vi "主程序.vi"() -> ()   [LabVIEW 2016]
panel:
  out "数值":dbl
  out "布尔":bool
  out "数字(0-1)":dbl
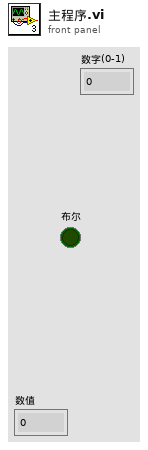
[diagram p1: front panel]
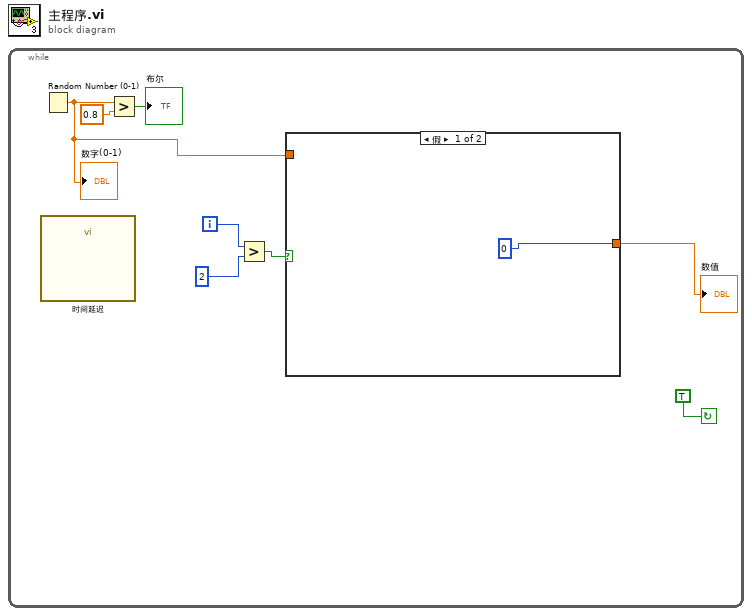
[diagram p0: block diagram]
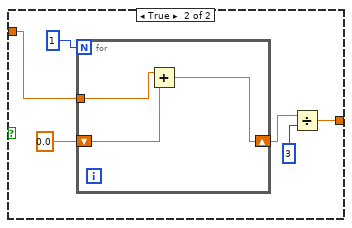
[diagram p2: hidden frame]
diagram:
  n1 = while {
    i -> [w2]
    stop <- TRUE continue-if-true
    n2 = call "时间延迟"() -> ()  [unwired: 11 in, 1 out]
    n3 = Random Number (0-1)() -> (number: 0 to 1=w5:dbl)
    "数字(0-1)" <- w5
    n4 = Greater?(x=w5, y=0.8) -> (0:→"布尔":bool)
    n5 = Greater?(x=w2, y=2) -> (0:w3:bool)
    n6 = case shown="假" w3 {
      tunnel: w5 -> [_ w15]
      tunnel: [0 w12] -> w4
      frame False {
      }
      frame True {
        n7 = for {
          N: 1 -> [_]
          tunnel: w15 -> [w18]
          shift-right: [w16] -> w10
          shift-left: 0.0 -> [w17]
          n8 = Add(x=w18, y=w17) -> (x+y=w16:dbl)
        }
        n9 = Divide(x=w10, y=3) -> (x/y=w12:dbl)
      }
    }
    "数值" <- w4
  }
